vi "PadCaseStructure.vi"(8 "error in (no error)":errorcluster, 11 "Bounding box for items in":T1) -> (0 "error out":errorcluster, 2 "Offset for items from outer top left corner":cluster{"Horizontal":i32, "Vertical":i32}, 3 "Padded bounding box for items":T1)   [LabVIEW 2017, in "ErrorStructureDrawer.lvlib"]
doc: "Add extra space to a bounding box for the items that we will be put inside a case structure, in order to calculate the necessary outer dimensions of that case structure. Extra space is required to account for: the case structure's border thickness, the size of its selected case field, and any desired whitespace."
uses:
  ErrorStructureDrawer.lvlib
  <vilib>/Utility/miscctls.llb/LVBoundsTypeDef.ctl
  GetErrorStructureConstants.vi
  GetErrorStructureInnerWhitespace.vi
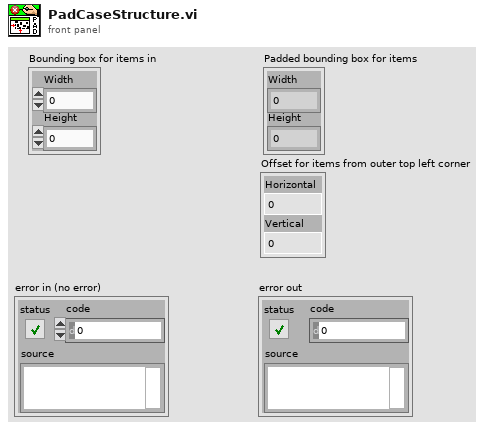
[diagram p1: front panel]
types:
  T1 = typedef "LVBoundsTypeDef.ctl" = cluster{"Width":u32, "Height":u32}
  T2 = typedef "ErrorStructureDrawer.lvlib/CaseStructureConstants.ctl" = cluster{"Border thickness":u32, "Case-menu height":u32, "Half height/width of a tunnel":i32}
  T3 = typedef "ErrorStructureDrawer.lvlib/CaseStructureInnerWhitespace.ctl" = cluster{"Left":u32, "Right":u32, "Top":u32, "Bottom":u32}
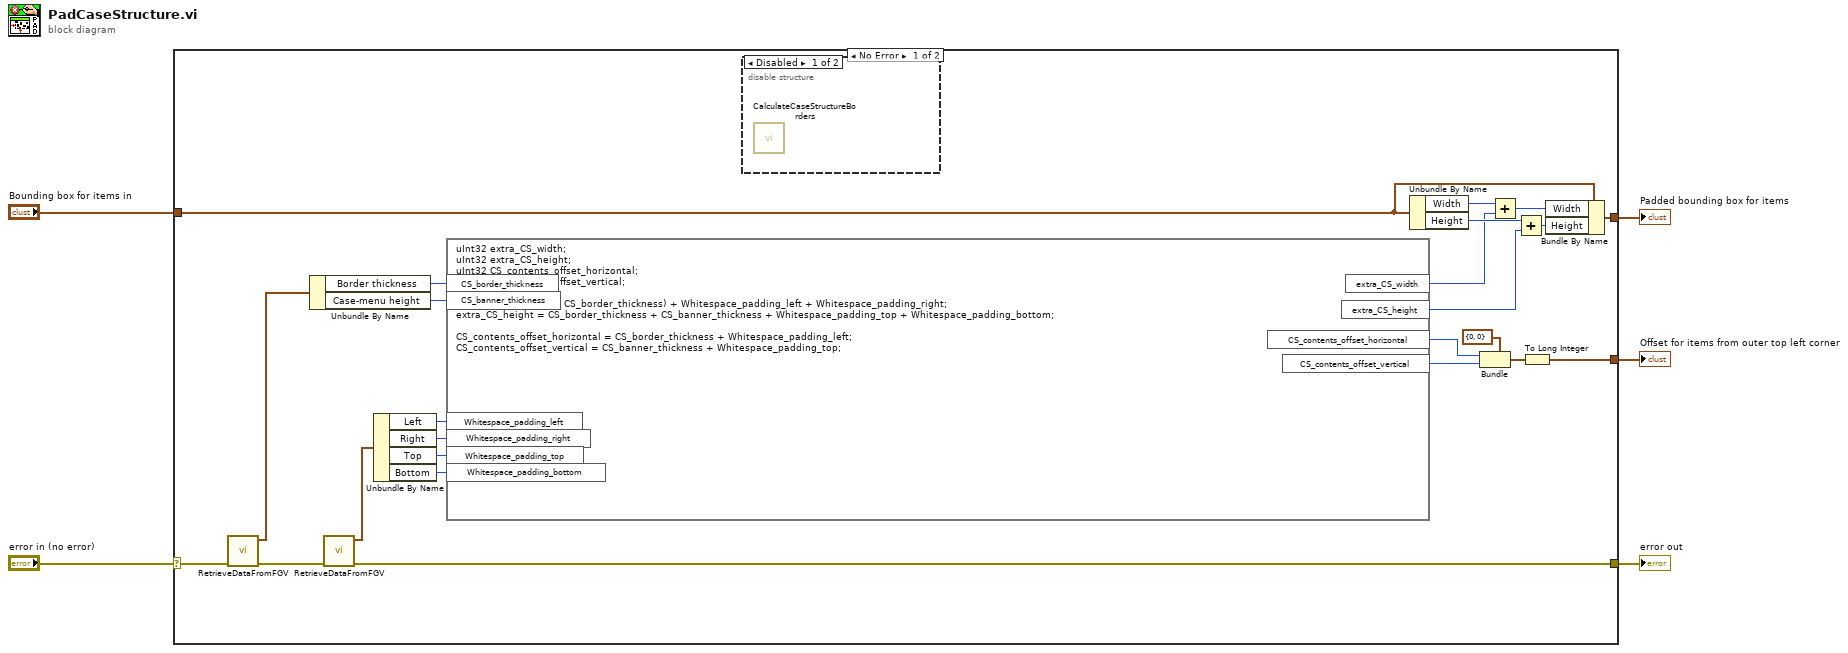
[diagram p0: block diagram]
diagram:
  n1 = case shown="No Error" "error in (no error)" {
    selector: "error in (no error)" -> [w10 w31]
    tunnel: "Bounding box for items in" -> [w29 w30]
    tunnel: [w28 w30] -> w4
    tunnel: [w17 _] -> w3
    tunnel: [w16 w31] -> w1
    frame No Error {
      n2 = call-poly "RetrieveDataFromFGV.vi"("error in (no error)"=w10) -> ("error out"=w9:errorcluster, "Case structure constants"=w8:T2)  [unwired: 9 in]
      n3 = Unbundle By Name(w8) -> ("Border thickness"=w7:u32, "Case-menu height"=w6:u32)
      n4 = call-poly "RetrieveDataFromFGV.vi"("error in (no error)"=w9) -> ("error out"=w16:errorcluster, "Case structure inner whitespace (px)"=w15:T3)  [unwired: 9 in]
      n5 = Unbundle By Name(w15) -> ("Left"=w11:u32, "Right"=w12:u32, "Top"=w13:u32, "Bottom"=w14:u32)
      n6 = formula code="uInt32 extra_CS_width;\nuInt32 extra_CS_height;\nuInt32 CS_contents_offset_horizontal;\nuInt32 CS_contents_offset_vertical;\n\nextra_CS_width = (2 * CS_border_thickness) + Whitespace_padding_left + Whitespace_padding_right;\nextra_CS_height = CS_border_thickness + CS_banner_thickness + Whitespace_padding_top + Whitespace_padding_bottom;\n\nCS_contents_offset_horizontal = CS_border_thickness + Whitespace_padding_left;\nCS_contents_offset_vertical = CS_banner_thickness + Whitespace_padding_top;"("CS_border_thickness"=w7, "CS_banner_thickness"=w6, "Whitespace_padding_left"=w11, "Whitespace_padding_right"=w12, "Whitespace_padding_top"=w13, "Whitespace_padding_bottom"=w14) -> ("extra_CS_width"=w23:u32, "extra_CS_height"=w22:u32, "CS_contents_offset_horizontal"=w20:u32, "CS_contents_offset_vertical"=w21:u32)
      n7 = disable-structure shown="Disabled" {
        frame Disabled {
          n8 = call "CalculateCaseStructureBorders.vi"() -> ()  [unwired: 11 in, 1 out]
        }
        frame Enabled {
        }
      }
      n9 = Unbundle By Name(w29) -> ("Width"=w25:u32, "Height"=w26:u32)
      n10 = Bundle(cluster=cluster{"Horizontal":u32, "Vertical":u32} {"Horizontal"=0, "Vertical"=0} ("Offsets"), "Horizontal"=w20, "Vertical"=w21) -> (w18:cluster{"Horizontal":u32, "Vertical":u32})
      n11 = Add(x=w25, y=w23) -> (x+y=w24:u32)
      n12 = Add(x=w26, y=w22) -> (x+y=w27:u32)
      n13 = To Long Integer(number=w18) -> (32bit integer=w17:cluster{"Horizontal":i32, "Vertical":i32})
      n14 = Bundle By Name(cluster=w29, "Width"=w24, "Height"=w27) -> (w28:T1)
    }
    frame Error {
    }
  }
  "Padded bounding box for items" <- w4
  "Offset for items from outer top left corner" <- w3
  "error out" <- w1
